vi "AnemoASCIIConversion.vi"(1 "Input string (from RS232)":string) -> (0 "Data out":T1)   [LabVIEW 2018]
uses:
  Clusters/AnemometerData.ctl
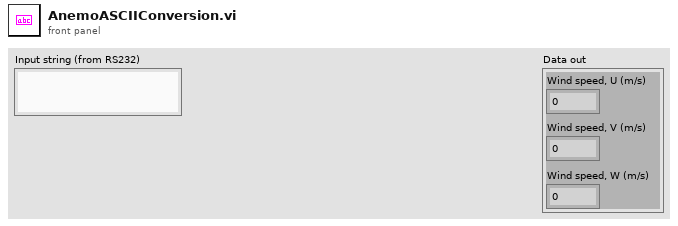
[diagram p1: front panel]
types:
  T1 = typedef "AnemometerData.ctl" = cluster{"Wind speed, U (m/s)":dbl, "Wind speed, V (m/s)":dbl, "Wind speed, W (m/s)":dbl}
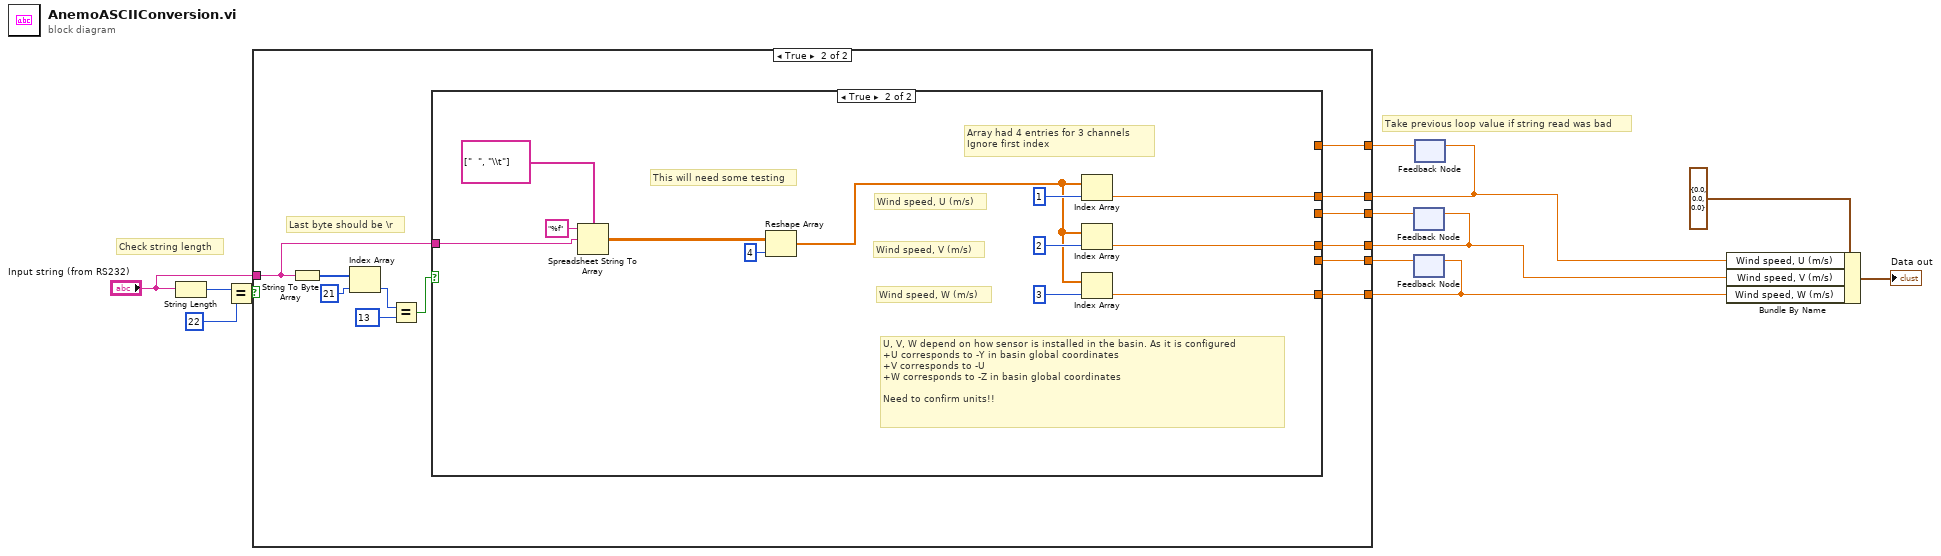
[diagram p0: block diagram]
diagram:
  # "Check string length"
  # "Take previous loop value if string read was bad"
  n1 = String Length(string="Input string (from RS232)") -> (length=w12:i32)
  n2 = Equal?(x=w12, y=22) -> (x = y?=w10:bool)
  n3 = feedback #1() -> (w7:dbl)  [unwired: 1 in]
  n4 = feedback #2() -> (w6:dbl)  [unwired: 1 in]
  n5 = feedback #3() -> (w8:dbl)  [unwired: 1 in]
  n6 = case shown="True" w10 {
    tunnel: [w13 w27] -> w2
    tunnel: [w14 w26] -> w3
    tunnel: [w15 w25] -> w4
    tunnel: "Input string (from RS232)" -> [_ w19]
    tunnel: w8 -> [w15 w18]
    tunnel: w7 -> [w14 w17]
    tunnel: w6 -> [w13 w16]
    frame False {
    }
    frame True {
      # "Last byte should be \\r"
      n7 = String To Byte Array(string=w19) -> (unsigned byte array=w23:u8[])
      n8 = Index Array(array=w23, index=21) -> (element=w22:u8)
      n9 = Equal?(x=w22, y=u8 13) -> (x = y?=w20:bool)
      n10 = case shown="True" w20 {
        tunnel: [w28 w34] -> w27
        tunnel: [w29 w33] -> w26
        tunnel: [w30 w32] -> w25
        tunnel: w19 -> [_ w31]
        tunnel: w18 -> [w30 _]
        tunnel: w17 -> [w29 _]
        tunnel: w16 -> [w28 _]
        frame False {
        }
        frame True {
          # "Array had 4 entries for 3 channels\nIgnore first index"
          # "U, V, W depend on how sensor is installed in the basin. As it is configured\n+U corresponds to -Y in basin global coordinates\n+V corresponds to -U\n+W corresponds to -Z in basin global coordinates \n\nNeed to confirm units!!"
          # "Wind speed, W (m/s)"
          # "Wind speed, V (m/s)"
          # "Wind speed, U (m/s)"
          # "This will need some testing"
          n11 = Spreadsheet String To Array(delimiter (Tab)=string[] ["  ", "\\t"], format string="%f", spreadsheet string=w31) -> (array=w41:dbl[][])  [unwired: 1 in]
          n12 = Reshape Array(w41, 4 ("dimension size")) -> (w35:dbl[])
          n13 = Index Array(array=w35, index=1) -> (element=w32:dbl)
          n14 = Index Array(array=w35, index=2) -> (element=w33:dbl)
          n15 = Index Array(array=w35, index=3) -> (element=w34:dbl)
        }
      }
    }
  }
  n16 = feedback-in #1(w3) -> ()
  n17 = feedback-in #2(w2) -> ()
  n18 = feedback-in #3(w4) -> ()
  n19 = Bundle By Name(cluster=T1 {"Wind speed, U (m/s)"=0.0, "Wind speed, V (m/s)"=0.0, "Wind speed, W (m/s)"=0.0} ("Data In"), "Wind speed, U (m/s)"=w4, "Wind speed, V (m/s)"=w3, "Wind speed, W (m/s)"=w2) -> (→"Data out":T1)
